vi "DB Insert.vi"(6 "Schema Name":string, 7 "Data":string[][](array[string]), 8 "error in (no error)":errorcluster, 9 "columns":string[](array[string]), 10 "table":string, 11 "Database in":refnum<class "MYSQL Database.lvclass">) -> (0 "error out":errorcluster, 2 "SQL":string caption="SQL+ (Col[]) VALUES (?[])", 3 "Database out":refnum<class "MYSQL Database.lvclass">)   [LabVIEW 2023, in "HardwareAbstractionLayer_LVOOP.lvlib" / "MYSQL Database.lvclass"]
doc: "This VI is DB SQL Insert Query"
uses:
  MYSQL Database.lvclass
  MYSQL Database.lvclass/MYSQL Database.ctl
  <vilib>/addons/database/Connection.llb/Conn Execute.vi
  <vilib>/addons/database/Recordset.llb/Rec Destroy - Connection.vi
  Database.lvclass
  <vilib>/addons/database/NI_Database_API.lvlib
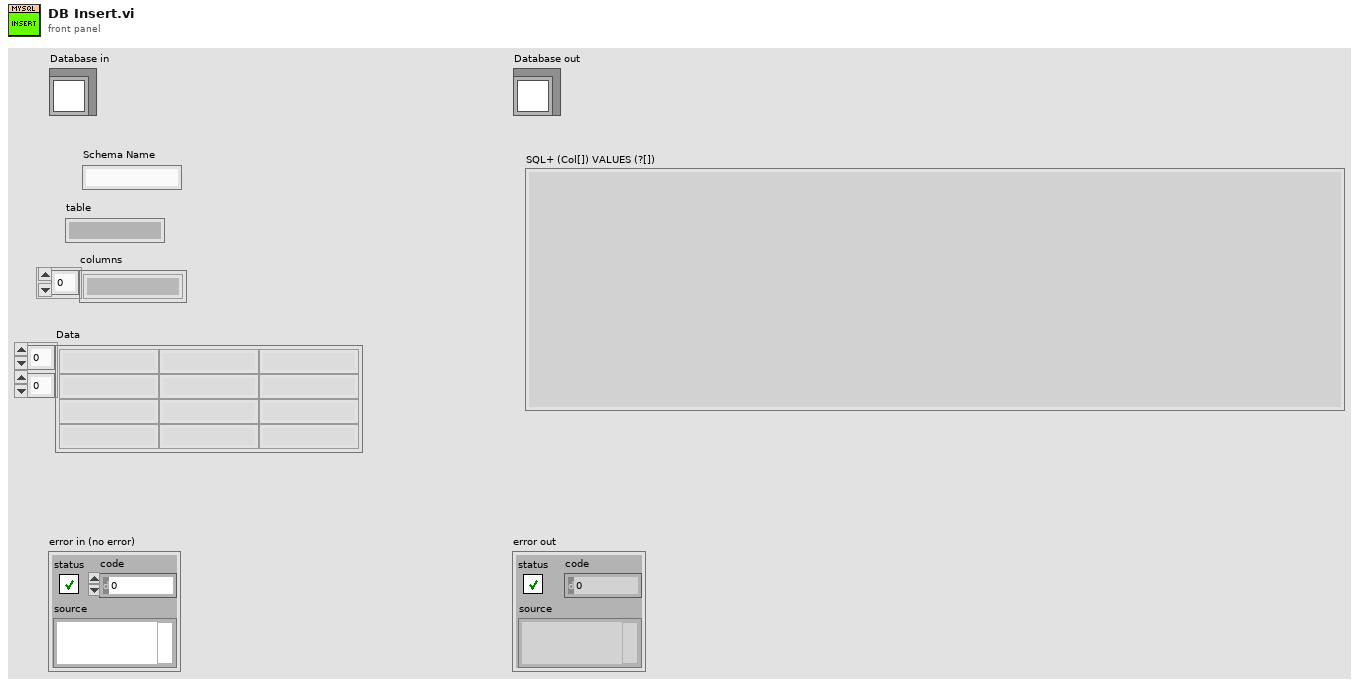
[diagram p1: front panel]
types:
  T1 = typedef "NI_Database_API.lvlib/Conn ObjectReference.ctl" = refnum<k1>
  T2 = typedef "NI_Database_API.lvlib/Rec ObjectReference.ctl" = refnum<k1>
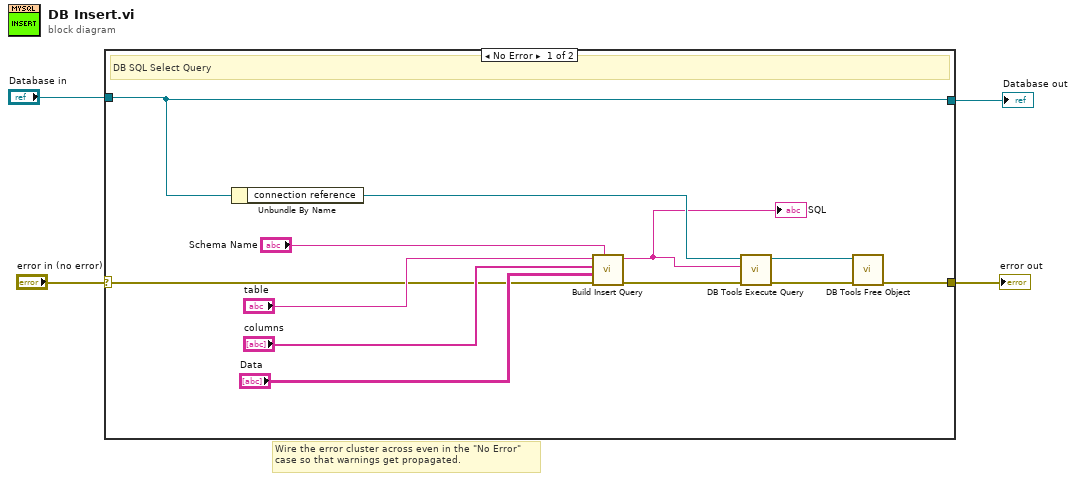
[diagram p0: block diagram]
diagram:
  # "Wire the error cluster across even in the \"No Error\"\ncase so that warnings get propagated."
  n1 = case shown="No Error" "error in (no error)" {
    selector: "error in (no error)" -> [w10 w18]
    tunnel: [w6 w18] -> w3
    tunnel: [w16 w17] -> w1
    tunnel: "Database in" -> [w16 w17]
    frame No Error {
      # "DB SQL Select Query"
      n2 = Unbundle By Name(w16) -> ("connection reference"=w12:T1)
      n3 = call "Build Insert Query.vi"("Schema Name"="Schema Name", "error in (no error)"=w10, "Data"="Data", "Column Names"="columns", "Table Name"="table") -> ("error out"=w9:errorcluster, "SQL"=w11:string)  [unwired: 5 in]
      "SQL" <- w11
      n4 = call-poly <vilib>:"DB Tools Execute Query.vi"("error in (no error)"=w9, "SQL query"=w11, "connection reference"=w12) -> ("error out"=w7:errorcluster, "recordset reference"=w8:T2)  [unwired: 5 in]
      n5 = call-poly <vilib>:"DB Tools Free Object.vi"("error in (no error)"=w7, "recordset reference"=w8) -> ("error out"=w6:errorcluster)  [unwired: 8 in, 1 out]
    }
    frame Error {
    }
  }
  "error out" <- w3
  "Database out" <- w1
